vi "Start Live.vi"(7 "Error In":errorcluster, 8 "Gain in":i32 min=0 max=2000 step=1, 9 "Exposure time (ms)":dbl, 10 "Camera reference in":refnum<k24>) -> (0 "Error Out":errorcluster, 3 "Camera reference out":refnum<k24>)   [LabVIEW 2017]
uses:
  C:/Program Files/National Instruments/LabVIEW 2017/instr.lib/IDS/ueye.NET/uEyeDotNet.dll
panel:
  out "Array":u16[][](array[numeric])
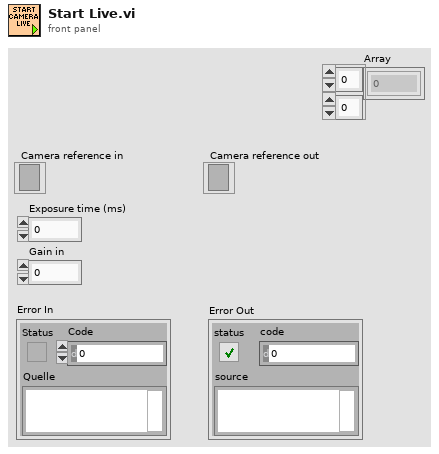
[diagram p1: front panel]
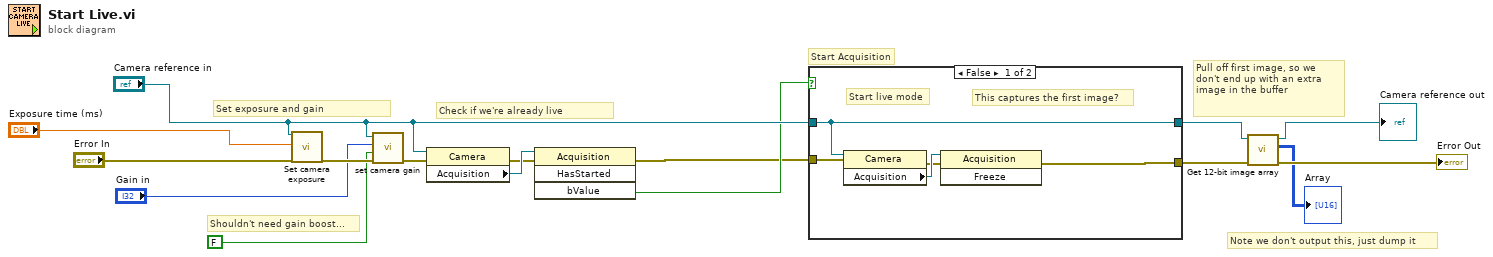
[diagram p0: block diagram]
diagram:
  # "Note we don't output this, just dump it"
  # "Pull off first image, so we don't end up with an extra image in the buffer"
  # "Set exposure and gain"
  # "Check if we're already live"
  # "Start Acquisition"
  # "Shouldn't need gain boost..."
  n1 = call "Set camera exposure.vi"("Camera reference in"="Camera reference in", "Exposure time (ms)"="Exposure time (ms)", "Error In"="Error In") -> ("Error Out"=w13:errorcluster)  [unwired: 15 in, 1 out]
  n2 = call "set camera gain.vi"("Error In"=w13, "Gain Boost in"=FALSE, "Gain in"="Gain in", ".NET (Reference)"="Camera reference in") -> ("Error Out"=w12:errorcluster)  [unwired: 5 in, 2 out]
  n3 = property class="Camera"(reference="Camera reference in", error in=w12) -> (error out=w7:errorcluster, "Acquisition"=w8:refnum<k24>)  [unwired: 1 out]
  n4 = invoke class="Acquisition" method="HasStarted"(reference=w8, error in=w7) -> (error out=w1:errorcluster, "bValue"=w9:bool)  [unwired: 2 in, 2 out]
  n5 = case shown="False" w9 {
    tunnel: [w17 w23] -> w6
    tunnel: w1 -> [w19 w23]
    tunnel: "Camera reference in" -> [w18 w22]
    tunnel: [w18 w22] -> w5
    frame False {
      # "This captures the first image?"
      # "Start live mode"
      n6 = property class="Camera"(reference=w18, error in=w19) -> (error out=w20:errorcluster, "Acquisition"=w21:refnum<k24>)  [unwired: 1 out]
      n7 = invoke class="Acquisition" method="Freeze"(reference=w21, error in=w20) -> (error out=w17:errorcluster)  [unwired: 1 in, 2 out]
    }
    frame True {
      # "We're already live"
    }
  }
  n8 = call "Get 12-bit image array.vi"("Error In"=w6, "Camera reference in"=w5) -> ("Error Out"=→"Error Out":errorcluster, "Array"=→"Array":u16[][], "Camera reference out"=→"Camera reference out":refnum<k24>)  [unwired: 6 in]
